vi "Refresh_List.vi"(6 "Code Type":T1, 7 "List":string[](array[string]), 8 "error in (no error)":errorcluster, 11 "Ref In":T2={"MS SQL Connection"=refnum, "UDL File"=path "", "Time"="", "DCODE"="", "WIP+1"=0, "MC No?"=0, "POKAYOKE?"=FALSE, "Expected Result"="", "Result [Status]"="", "Clock"=0.0, "RFID"="", "WIP Queue"=refnum, "TS Parameter"={"ProfitCenterCode"="", "LineCode"="", "WorkOrderNumber"="", "Model"="", "Model_with_Prefix"="", "VendorCode"="", "SetParameterDateCode"="", "PokaYoke"=0, "Target"=1, "Live_DateCode"="", "CustomerPartNumber"="", "Hand"="", "sBarcode"=FALSE, "FCA"=0, "Ent_Stamp"=timestamp(0 s since 1904-01-01), "STS_CD"=0.0}, "Data_Queue"=[], "RFID Serial No."=""} {"TS Parameter"."FCA" format="%01d"; "TS Parameter"."Target" min=1 max=100000; "TS Parameter"."PokaYoke" min=0 max=1}) -> (0 "error out":errorcluster)   [LabVIEW 2020]
uses:
  Controls/TD SQL.ctl
  <vilib>/addons/database/Connection.llb/Conn ObjectReference.ctl
  Controls/WIP_State.ctl
  Controls/TS_Parameter.ctl
  Controls/Loss_type.ctl
  <vilib>/addons/database/NI_Database_API.lvlib
panel:
  out "spreadsheet string":string
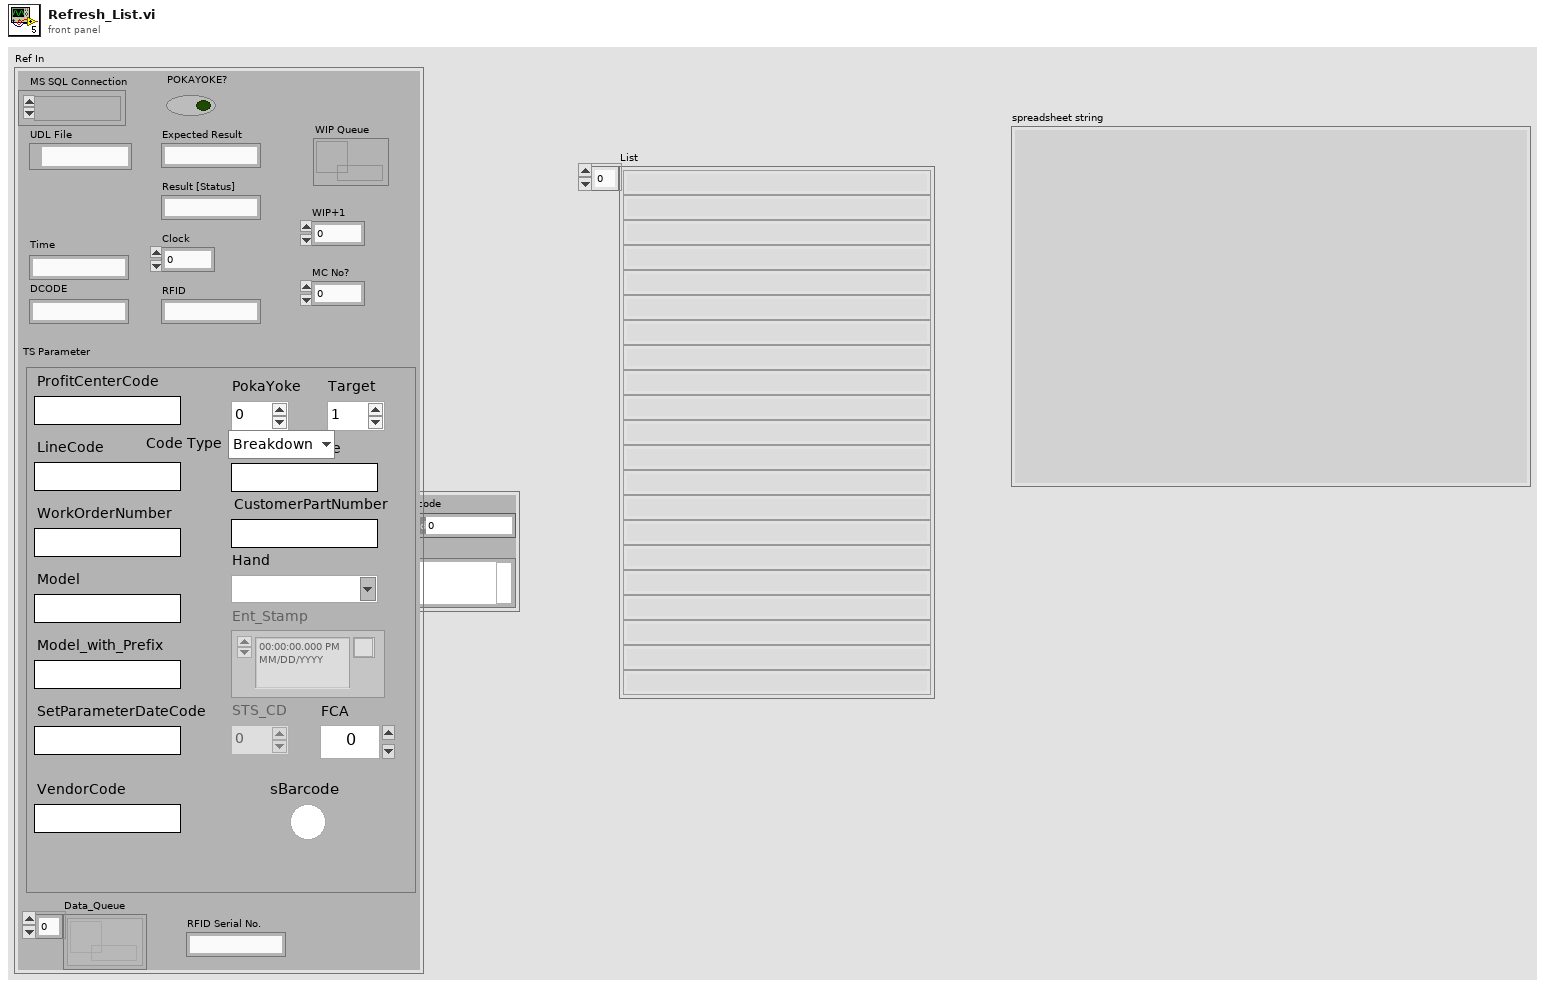
[diagram p1: front panel]
types:
  T1 = typedef "Loss_type.ctl" = enum16{"Breakdown", "Bookout"}
  T2 = typedef "TD SQL.ctl" = cluster{"MS SQL Connection":T3, "UDL File":path, "Time":string, "DCODE":string, "WIP+1":i64, "MC No?":i32, "POKAYOKE?":bool, "Expected Result":string, "Result [Status]":string, "Clock":dbl, "RFID":string, "WIP Queue":refnum<queue>, "TS Parameter":T4, "Data_Queue":refnum<queue>[], "RFID Serial No.":string}
  T3 = typedef "NI_Database_API.lvlib/Conn ObjectReference.ctl" = refnum<k1>
  T4 = typedef "TS_Parameter.ctl" = cluster{"ProfitCenterCode":string, "LineCode":string, "WorkOrderNumber":string, "Model":string, "Model_with_Prefix":string, "VendorCode":string, "SetParameterDateCode":string, "PokaYoke":i32, "Target":i32, "Live_DateCode":string, "CustomerPartNumber":string, "Hand":string, "sBarcode":bool, "FCA":i32, "Ent_Stamp":timestamp, "STS_CD":dbl}
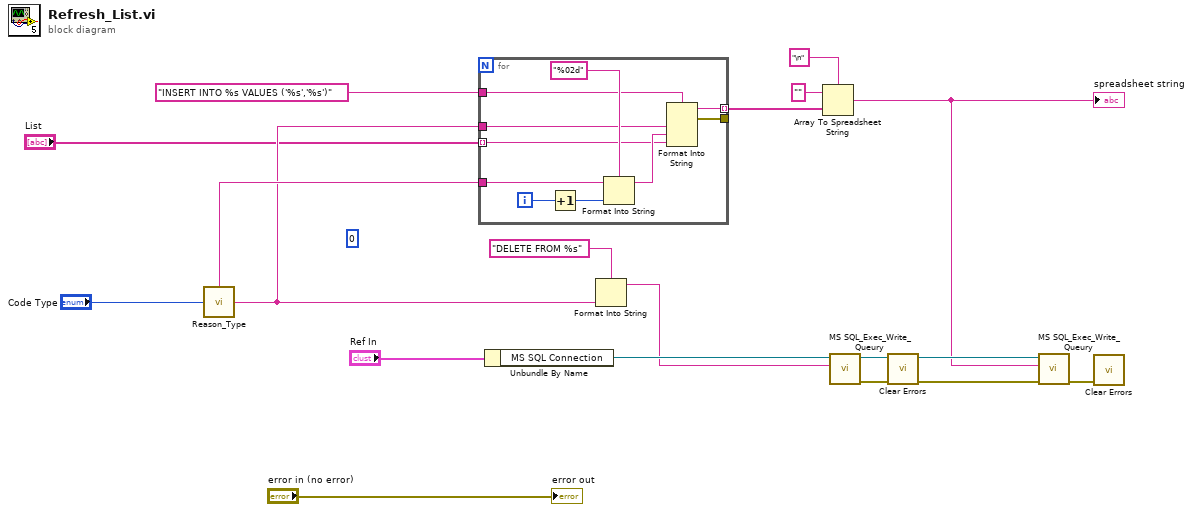
[diagram p0: block diagram]
diagram:
  (unwired) 0
  n1 = call "Reason_Type.vi"("Reason Type"="Code Type") -> ("Break|Bookout"=w11:string, "Hint"=w13:string)  [unwired: 2 in]
  n2 = for {
    tunnel: "List" -> [w19] mode=indexing
    tunnel: w13 -> [w26]
    tunnel: "INSERT INTO %s VALUES ('%s','%s')" ("trimmed string") -> [w24]
    tunnel: w11 -> [w23]
    tunnel: [w21] -> w10 mode=indexing
    tunnel: [w20] -> _
    i -> [w27]
    n3 = Increment(x=w27) -> (x+1=w25:i32)
    n4 = Format Into String(format string="%02d", initial string=w26, w25) -> (resulting string=w22:string)  [unwired: 1 in, 1 out]
    n5 = Format Into String(format string=w24, w23, w22, w19) -> (resulting string=w21:string, error out=w20:errorcluster)  [unwired: 2 in]
  }
  n6 = Unbundle By Name("Ref In") -> ("MS SQL Connection"=w16:T3)
  n7 = Format Into String(format string="DELETE FROM %s" ("Query"), w11) -> (resulting string=w14:string)  [unwired: 2 in, 1 out]
  n8 = Array To Spreadsheet String(delimiter (Tab)="\n", array=w10, 3:"" ("format string")) -> (spreadsheet string=w5:string)
  "spreadsheet string" <- w5
  n9 = call "MS SQL_Exec_Write_Queury.vi"("Query"=w14, "Refnum in"=w16) -> ("error out"=w7:errorcluster, "Refnum out"=w6:T3)  [unwired: 8 in]
  n10 = call <vilib>:"Clear Errors.vi"("error in (no error)"=w7) -> ("error out"=w3:errorcluster)  [unwired: 5 in, 1 out]
  n11 = call "MS SQL_Exec_Write_Queury.vi"("error in (no error)"=w3, "Query"=w5, "Refnum in"=w6) -> ("error out"=w2:errorcluster)  [unwired: 7 in, 1 out]
  n12 = call <vilib>:"Clear Errors.vi"("error in (no error)"=w2) -> ()  [unwired: 5 in, 2 out]
  "error out" <- "error in (no error)"
